vi "subGetItemType.vi"(9 "Property value":string, 11 "Refnum in":refnum<k20>) -> (3 "Nodes":refnum<k20>[](array[refnum]))   [LabVIEW 2020, in "SolutionBuilder.lvlib"]
uses:
  SolutionBuilder.lvlib
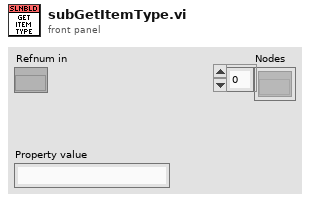
[diagram p1: front panel]
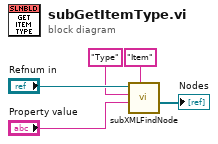
[diagram p0: block diagram]
diagram:
  n1 = call "subXMLFindNode.vi"("Node name"="Item", "Property value"="Property value", "Property name"="Type", "Refnum in"="Refnum in") -> ("Nodes"=→"Nodes":refnum<k20>[])  [unwired: 6 in, 1 out]
